vi "BUZZER AND IR SENSOR.vi"() -> ()   [LabVIEW 2018]
uses:
  <vilib>/DAQmx/read.llb/DAQmx Read (Digital Bool 1Line 1Point).vi
  <vilib>/DAQmx/write.llb/DAQmx Write (Digital 1D Bool NChan 1Samp 1Line).vi
  <vilib>/DAQmx/create/channels.llb/DAQmx Create Channel (DO-Digital Output).vi
  <vilib>/DAQmx/create/channels.llb/DAQmx Create Channel (DI-Digital Input).vi
  <vilib>/DAQmx/miscellaneous.llb/DAQmx Fill In Error Info.vi
panel:
  in  "s":bool
  out "Numeric":dbl
  out "data 2":bool
  in  "stop":bool
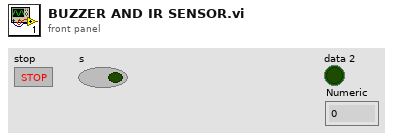
[diagram p1: front panel]
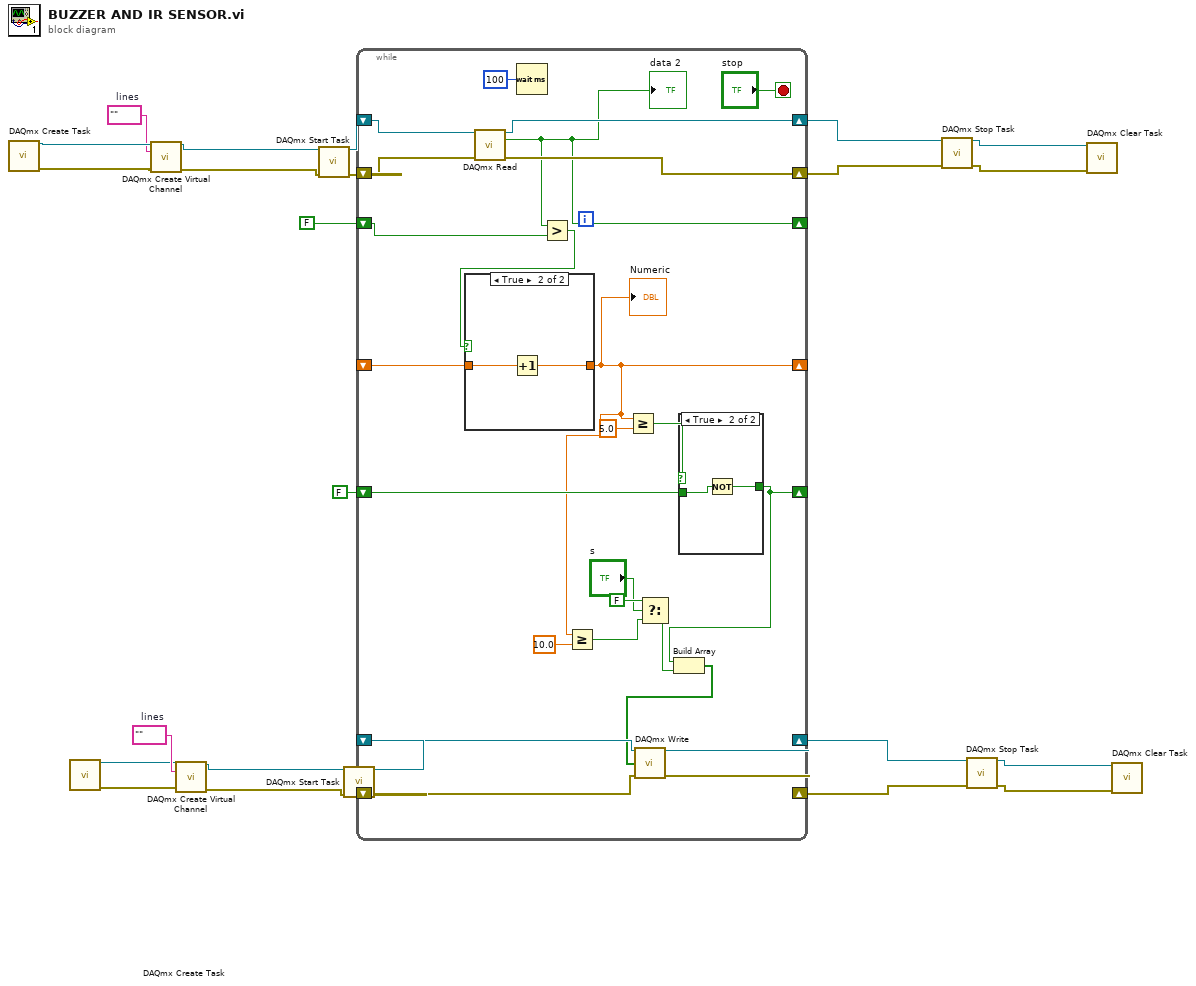
[diagram p0: block diagram]
diagram:
  w12 = tag ""  # lines
  w15 = tag ""  # lines
  n1 = call <vilib>:"DAQmx Create Task.vi"() -> ("task out"=w13:refnum<k21>, "error out"=w11:errorcluster)  [unwired: 14 in]
  n2 = call <vilib>:"DAQmx Create Task.vi"() -> ("task out"=w14:refnum<k21>, "error out"=w16:errorcluster)  [unwired: 14 in]
  n3 = call-poly <vilib>:"DAQmx Create Virtual Channel.vi"("task in"=w13, "lines"=w12, "error in"=w11) -> ("task out"=w10:refnum<k21>, "error out"=w9:errorcluster)  [unwired: 11 in]
  n4 = call-poly <vilib>:"DAQmx Create Virtual Channel.vi"("task in"=w14, "lines"=w15, "error in"=w16) -> ("task out"=w17:refnum<k21>, "error out"=w18:errorcluster)  [unwired: 11 in]
  n5 = call <vilib>:"DAQmx Start Task.vi"("task/channels in"=w10, "error in"=w9) -> ("task out"=w8:refnum<k21>, "error out"=w7:errorcluster)  [unwired: 12 in]
  n6 = call <vilib>:"DAQmx Start Task.vi"("task/channels in"=w17, "error in"=w18) -> ("task out"=w19:refnum<k21>, "error out"=w20:errorcluster)  [unwired: 12 in]
  n7 = while {
    shift-right: [w46] -> w22
    shift-left: w19 -> [w44]
    shift-right: [w47] -> w24
    shift-left: w20 -> [w45]
    shift-right: [w41] -> w5
    shift-left: w8 -> [w43]
    shift-right: [w40] -> w3
    shift-left: w7 -> [w42]
    shift-right: [w37] -> _
    shift-left: FALSE -> [w36]
    shift-right: [w30] -> _
    shift-left: FALSE -> [w39]
    shift-right: [w27] -> _
    shift-left: _ -> [w35]
    stop <- "stop" stop-if-true
    n8 = call-poly <vilib>:"DAQmx Read.vi"("task/channels in"=w43, "error in"=w42) -> ("task out"=w41:refnum<k21>, "data"=w37:bool, "error out"=w40:errorcluster)  [unwired: 11 in]
    "data 2" <- w37
    n9 = Wait (ms)(milliseconds to wait=u32 100) -> ()  [unwired: 1 out]
    n10 = Greater?(x=w37, y=w36) -> (0:w38:bool)
    n11 = case shown="True" w38 {
      tunnel: [w53 w55] -> w27
      tunnel: w35 -> [w53 w54]
      frame False {
      }
      frame True {
        n12 = Increment(x=w54) -> (x+1=w55:dbl)
      }
    }
    "Numeric" <- w27
    n13 = Greater Or Equal?(x=w27, y=10.0) -> (x >= y?=w33:bool)
    n14 = Greater Or Equal?(x=w27, y=5.0) -> (x >= y?=w25:bool)
    n15 = Select(t=FALSE, s="s", f=w33) -> (s? t:f=w29:bool)
    n16 = case shown="True" w25 {
      tunnel: w39 -> [w50 w52]
      tunnel: [w50 w51] -> w30
      frame False {
      }
      frame True {
        n17 = Not(x=w52) -> (.not. x?=w51:bool)
      }
    }
    n18 = Build Array(w30, w29) -> (w26:bool[])
    n19 = call-poly <vilib>:"DAQmx Write.vi"("task/channels in"=w44, "data"=w26, "error in"=w45) -> ("task out"=w46:refnum<k21>, "error out"=w47:errorcluster)  [unwired: 10 in, 1 out]
  }
  n20 = call <vilib>:"DAQmx Stop Task.vi"("task/channels in"=w5, "error in"=w3) -> ("task out"=w6:refnum<k21>, "error out"=w4:errorcluster)  [unwired: 12 in]
  n21 = call <vilib>:"DAQmx Stop Task.vi"("task/channels in"=w22, "error in"=w24) -> ("task out"=w21:refnum<k21>, "error out"=w23:errorcluster)  [unwired: 12 in]
  n22 = call <vilib>:"DAQmx Clear Task.vi"("task in"=w6, "error in"=w4) -> ()  [unwired: 13 in, 1 out]
  n23 = call <vilib>:"DAQmx Clear Task.vi"("task in"=w21, "error in"=w23) -> ()  [unwired: 13 in, 1 out]
